vi "ISEG_HVSystemGUI.createObject.vi"(0 "Object name":string, 1 "Class name":string, 2 "constructor":string="constructor.vi", 3 "data":string, 4 "timeout (ms)":i32=10000, 5 "error in (no error)":errorcluster) -> (19 "error out":errorcluster)   [LabVIEW 2014, in "ISEG_HVSystemGUI.lvlib"]
uses:
  ISEG_HVSystemGUI.lvlib
  CS_Core/CSSystem/CoreDefs/CoreDefs.call_type.ctl
  CS_Core/BaseProcess/BaseProcess.descriptor string definition.ctl
  CS_Core/CSSystem/CoreDefs/CoreDefs.rawDataType.ctl
  CS_Core/CSSystem/CoreLib/CoreLib.string 2 byte array.vi
  CS_Core/CSSystem/CSSystemLib/CSSystemLib.lvlib
  CS_Core/CSSystem/CoreLib/CoreLib.lvlib
  CS_Core/BaseProcess/BaseProcess.lvlib
panel:
  in  "call cluster":T1
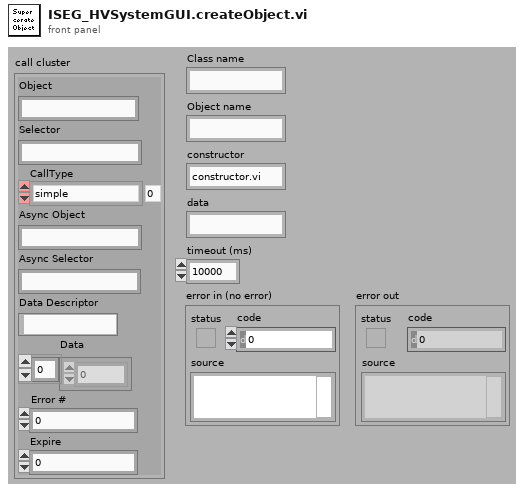
[diagram p1: front panel]
types:
  T1 = typedef "CoreDefs.call_type.ctl" = cluster{"Object":string, "Selector":string, "CallType":enum16{"simple", "synchronous", "asynchronous"}, "Async Object":string, "Async Selector":string, "Data Descriptor":T2, "Data":T3, "Error #":i32, "Expire":u32}
  T2 = typedef "BaseProcess.lvlib/BaseProcess.descriptor string definition.ctl" = string
  T3 = typedef "CoreDefs.rawDataType.ctl" = i8[]
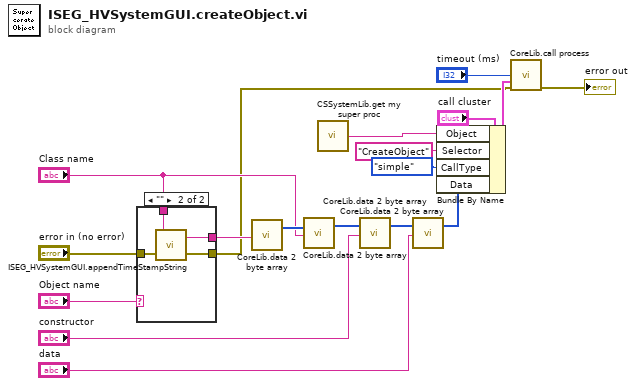
[diagram p0: block diagram]
diagram:
  n1 = case shown="\"\"" "Object name" {
    selector: "Object name" -> [w20 _]
    tunnel: "Class name" -> [_ w24]
    tunnel: [w20 w21] -> w4
    tunnel: [w19 w22] -> w3
    tunnel: "error in (no error)" -> [w19 w23]
    frame Default {
    }
    frame "" {
      n2 = call "ISEG_HVSystemGUI.appendTimeStampString.vi"("error in"=w23, "String"=w24) -> ("error out"=w22:errorcluster, "String with TS"=w21:string)
    }
  }
  n3 = call-poly "CoreLib.data 2 byte array.vi"("string"=w4) -> ("byteArray out"=w13:T3)  [unwired: 1 in, 17 out]
  n4 = call-poly "CoreLib.data 2 byte array.vi"("byteArray"=w13, "string"="Class name") -> ("byteArray out"=w14:T3)  [unwired: 17 out]
  n5 = call "CSSystemLib.get my super proc.vi"() -> ("name"=w12:string)  [unwired: 1 out]
  n6 = call-poly "CoreLib.data 2 byte array.vi"("byteArray"=w14, "string"="constructor") -> ("byteArray out"=w15:T3)  [unwired: 17 out]
  n7 = call-poly "CoreLib.data 2 byte array.vi"("byteArray"=w15, "string"="data") -> ("byteArray out"=w18:T3)  [unwired: 17 out]
  n8 = Bundle By Name(cluster="call cluster", "Object"=w12, "Selector"="CreateObject", "CallType"=enum16{"simple", "synchronous", "asynchronous"}."simple", "Data"=w18) -> (w11:T1)
  n9 = call "CoreLib.call process.vi"("timeout (ms)"="timeout (ms)", "call cluster in"=w11, "error in (no error)"=w3) -> ("error out"=→"error out":errorcluster)  [unwired: 1 in, 11 out]
